vi "Module Demo.vi"() -> ()   [LabVIEW 2011]
panel:
  out "Falling Edge":bool
  out "Numeric":i32
  in  "Boolean Input":bool
  in  "stop":bool
  out "Counter":i32
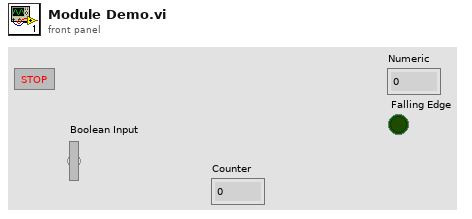
[diagram p1: front panel]
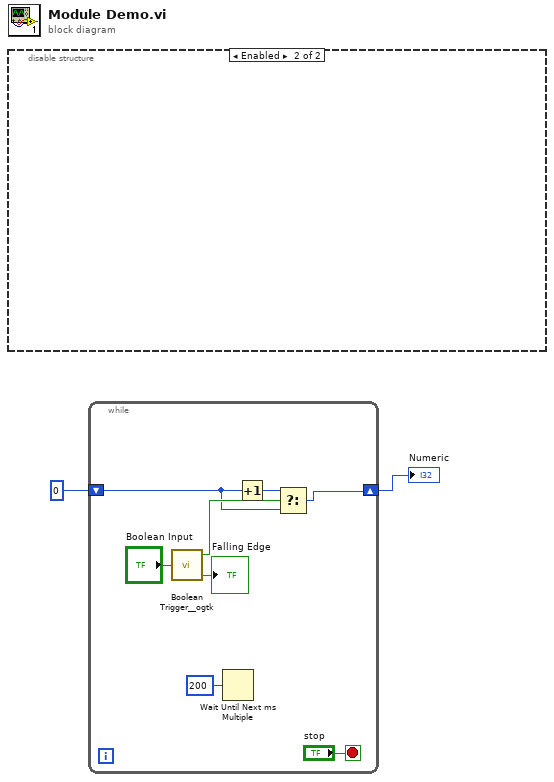
[diagram p0: block diagram]
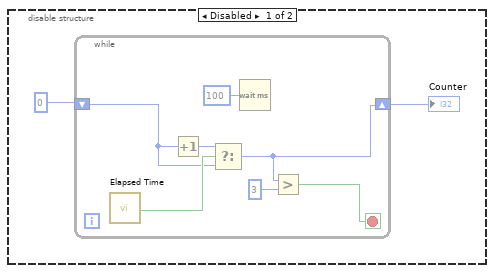
[diagram p2: hidden frame]
diagram:
  n1 = disable-structure shown="Enabled" {
    frame Disabled {
      n2 = while {
        shift-right: [w8] -> w3
        shift-left: 0 -> [w9]
        stop <- w6 stop-if-true
        n3 = call "Elapsed Time"() -> ("Time has Elapsed"=w11:bool)  [unwired: 12 in, 7 out]
        n4 = Increment(x=w9) -> (x+1=w10:i32)
        n5 = Select(t=w10, s=w11, f=w9) -> (s? t:f=w8:i32)
        n6 = Wait (ms)(milliseconds to wait=u32 100) -> ()  [unwired: 1 out]
        n7 = Greater?(x=w8, y=3) -> (0:w6:bool)
      }
      "Counter" <- w3
    }
    frame Enabled {
    }
  }
  n8 = while {
    shift-right: [w16] -> w1
    shift-left: 0 -> [w14]
    stop <- "stop" stop-if-true
    n9 = call <userlib>:"Boolean Trigger__ogtk.vi"("Boolean Input"="Boolean Input") -> ("Rising Edge"=w17:bool, "Falling Edge"=→"Falling Edge":bool)  [unwired: 1 in]
    n10 = Wait Until Next ms Multiple(millisecond multiple=u32 200) -> ()  [unwired: 1 out]
    n11 = Increment(x=w14) -> (x+1=w15:i32)
    n12 = Select(t=w15, s=w17, f=w14) -> (s? t:f=w16:i32)
  }
  "Numeric" <- w1
